vi "sm string read and increment.vi"(8 "Identifier":string="default", 11 "Shared memory cluster":T1) -> (2 "String out":string, 3 "Shared memory cluster output":T1)   [LabVIEW 2020, in "linuxSharedMemory.lvlib"]
uses:
  linuxSharedMemory.lvlib
  controls/sm_cluster.ctl
  <vilib>/NI/NI Linux RT IPC/Shared Memory/Pointer Operations/Read String.vi
  <vilib>/NI/NI Linux RT IPC/Shared Memory/Pointer Operations/In Place Read String.vi
  <vilib>/NI/NI Linux RT IPC/Shared Memory/Linux RT IPC.Shared Memory.lvlib
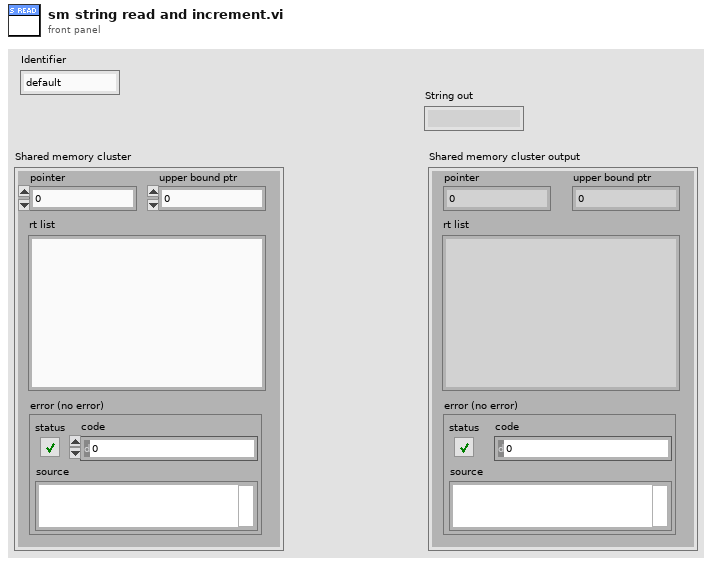
[diagram p1: front panel]
types:
  T1 = typedef "linuxSharedMemory.lvlib/sm_cluster.ctl" = cluster{"rt list":string, "error (no error)":errorcluster, "pointer":u64, "upper bound ptr":u64}
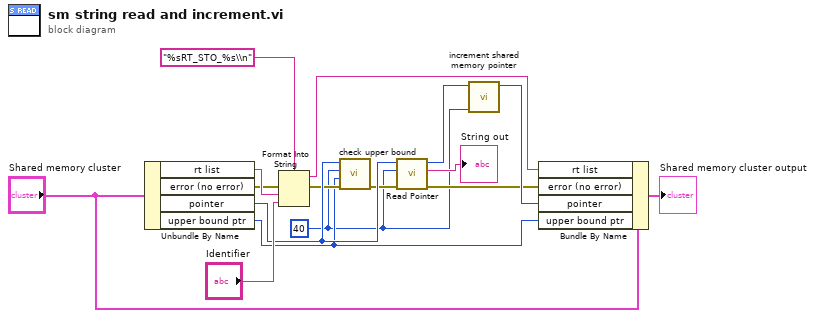
[diagram p0: block diagram]
diagram:
  w1 = u64 40
  n1 = Unbundle By Name("Shared memory cluster") -> ("rt list"=w14:string, "error (no error)"=w9:errorcluster, "pointer"=w8:u64, "upper bound ptr"=w3:u64)
  n2 = Format Into String(format string="%sRT_STO_%s\\n", error in=w9, w14, "Identifier") -> (resulting string=w11:string, error out=w7:errorcluster)  [unwired: 1 in]
  n3 = call "check upper bound.vi"("error in (no error)"=w7, "ptr upper bound (inclusive)"=w3, "size"=w1, "ptr in"=w8) -> ("error out"=w6:errorcluster)  [unwired: 7 in]
  n4 = call-poly <vilib>:"Read Pointer.vi"("error in (no error)"=w6, "bytes to read"=w1, "pointer in"=w8) -> ("error out"=w12:errorcluster, "string out"=→"String out":string, "pointer out"=w16:u64)  [unwired: 5 in, 1 out]
  n5 = call "increment shared memory pointer.vi"("Increment value"=w1, "Shared Memory PTR in"=w16) -> ("Shared Memory PTR out"=w13:u64)  [unwired: 9 in]
  n6 = Bundle By Name(cluster="Shared memory cluster", "rt list"=w11, "error (no error)"=w12, "pointer"=w13, "upper bound ptr"=w3) -> (→"Shared memory cluster output":T1)
